vi "create movie.vi"() -> ()   [LabVIEW 2012]
uses:
  <vilib>/vision/Avi.llb/IMAQ AVI2 Codec Path.ctl
panel:
  out "Codec Names":string[](array[string])
  in  "Image Folder Path":path
  in  "Frames Per Second":u32=30
  in  "AVI Path":path
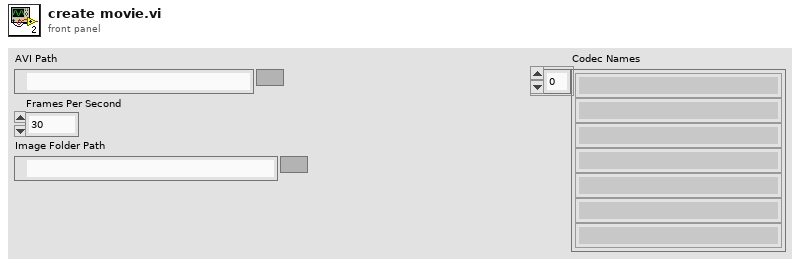
[diagram p1: front panel]
types:
  T1 = typedef "IMAQ AVI2 Codec Path.ctl" = u32
  T2 = typedef "IMAQ Image.ctl" = refnum<image>
  T3 = typedef "IMAQ AVI2 Refnum.ctl" = refnum<k20>
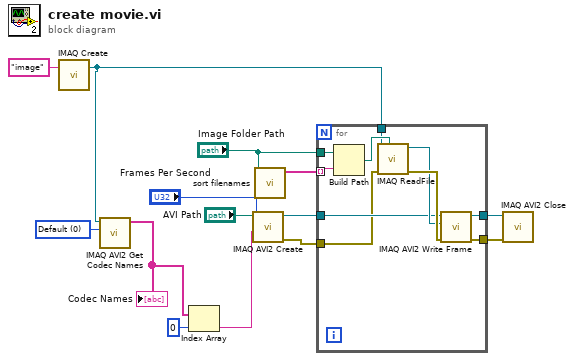
[diagram p0: block diagram]
diagram:
  w4 = T1 0 items=["Default", "System", "Built in Vision"] ("Codec Source")
  n1 = call "IMAQ Create"("Image Name"="image") -> ("New Image"=w5:T2)  [unwired: 4 in, 1 out]
  n2 = call "IMAQ AVI2 Get Codec Names"("Codec Source"=w4, "Image"=w5) -> ("Codec Names"=w3:string[])  [unwired: 8 in, 1 out]
  "Codec Names" <- w3
  n3 = Index Array(array=w3, index=0) -> (element=w1:string)
  n4 = call "IMAQ AVI2 Create"("Codec"=w1, "Frames Per Second"="Frames Per Second", "AVI Path"="AVI Path") -> ("error out"=w7:errorcluster, "AVI Refnum"=w10:T3)  [unwired: 7 in]
  n5 = call "sort filenames.vi"("Image Folder Path"="Image Folder Path") -> ("Sorted Names"=w12:string[])  [unwired: 10 in]
  n6 = for {
    tunnel: w12 -> [w20] mode=indexing
    tunnel: "Image Folder Path" -> [w21]
    tunnel: w10 -> [w19]
    tunnel: [w18] -> w9
    tunnel: [w17] -> w8
    tunnel: w7 -> [w16]
    tunnel: w5 -> [w15]
    n7 = Build Path(base path=w21, name or relative path=w20) -> (appended path=w22:path)
    n8 = call "IMAQ ReadFile"("File Path"=w22, "error in (no error)"=w16, "Image"=w15) -> ("error out"=w24:errorcluster, "Image Out"=w23:T2)  [unwired: 4 in, 3 out]
    n9 = call "IMAQ AVI2 Write Frame"("error in (no error)"=w24, "Image"=w23, "AVI Refnum"=w19) -> ("error out"=w17:errorcluster, "AVI Refnum (duplicate)"=w18:T3)  [unwired: 6 in, 1 out]
  }
  n10 = call "IMAQ AVI2 Close"("error in (no error)"=w8, "AVI Refnum"=w9) -> ()  [unwired: 9 in, 1 out]
